vi "Create.vi"(7 "Name":string) -> (8 "Channel":refnum<class "Channel.lvclass">)   [LabVIEW 2020, in "Channel.lvclass"]
uses:
  Channel.lvclass
  Channel.lvclass/Channel.ctl
  Level/Level.lvclass
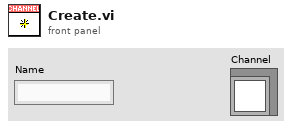
[diagram p1: front panel]
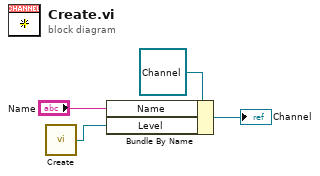
[diagram p0: block diagram]
diagram:
  n1 = call "Create.vi"() -> ("Level"=w1:refnum<class "Level.lvclass">)  [unwired: 15 in]
  n2 = Bundle By Name(cluster=refnum<class "Channel.lvclass"> refnum ("Channel"), "Name"="Name", "Level"=w1) -> (→"Channel":refnum<class "Channel.lvclass">)
